vi "FromJSON.vi"(8 "error in (no error)":errorcluster, 10 "Request":string) -> (0 "error out":errorcluster, 3 "Request out":refnum<class "Request.lvclass">)   [LabVIEW 2015, in "Request.lvclass"]
uses:
  Request.lvclass
  JsonCluster.ctl
  Request.lvclass/Request.ctl
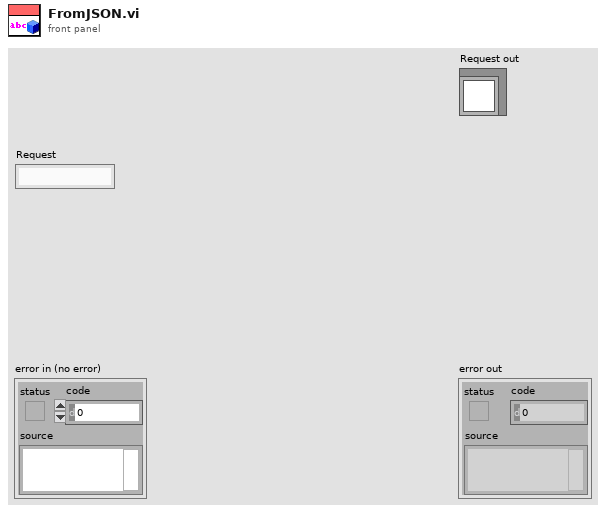
[diagram p1: front panel]
types:
  T1 = typedef "Request.lvclass/JsonCluster.ctl" = cluster{"RequestID":string, "PersonnelType":i32, "StartTime":string, "StartName":string, "AckTime":string, "AckName":string, "FulfilledTime":string, "FulfilledName":string, "Description":string, "RoomNumber":i32, "RequestType":i32, "Alarm":bool}
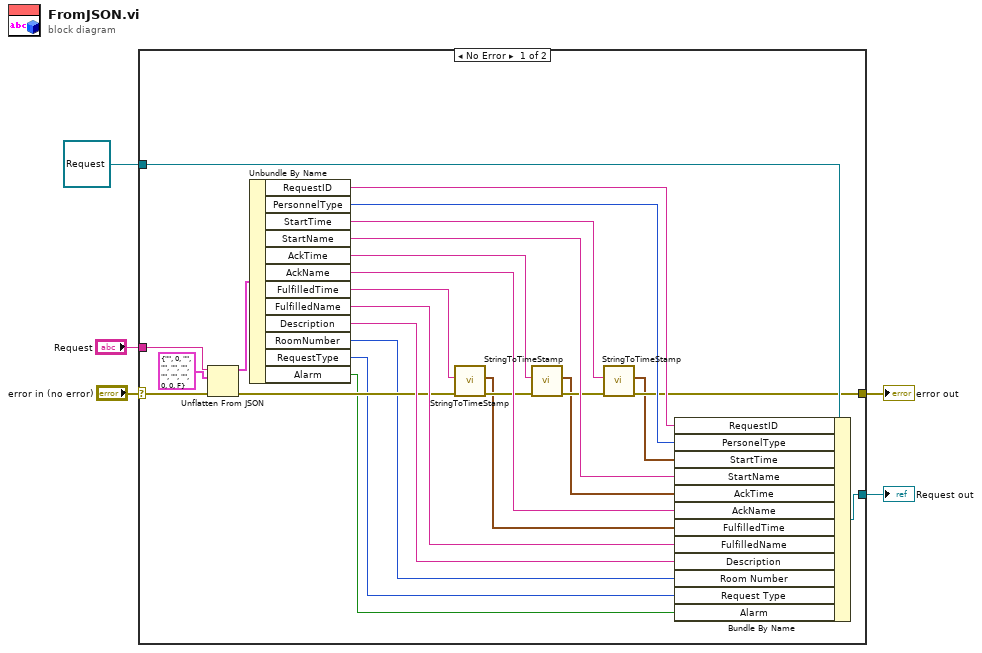
[diagram p0: block diagram]
diagram:
  n1 = case shown="No Error" "error in (no error)" {
    selector: "error in (no error)" -> [w16 w32]
    tunnel: [w17 w32] -> w4
    tunnel: [w29 w31] -> w2
    tunnel: refnum<class "Request.lvclass"> refnum ("Request in") -> [w30 w31]
    tunnel: "Request" -> [w28 _]
    frame No Error {
      n2 = Unflatten From JSON(JSON string=w28, type and defaults=T1 {"RequestID"="", "PersonnelType"=0, "StartTime"="", "StartName"="", "AckTime"="", "AckName"="", "FulfilledTime"="", "FulfilledName"="", "Description"="", "RoomNumber"=0, "RequestType"=0, "Alarm"=FALSE} ("RequestTable"), error in (no error)=w16) -> (value=w26:T1, error out=w15:errorcluster)  [unwired: 4 in]
      n3 = Unbundle By Name(w26) -> ("RequestID"=w25:string, "PersonnelType"=w20:i32, "StartTime"=w14:string, "StartName"=w21:string, "AckTime"=w12:string, "AckName"=w22:string, "FulfilledTime"=w10:string, "FulfilledName"=w23:string, "Description"=w24:string, "RoomNumber"=w8:i32, "RequestType"=w7:i32, "Alarm"=w6:bool)
      n4 = call "StringToTimeStamp.vi"("error in (no error)"=w15, "TimeStamp"=w10) -> ("error out"=w19:errorcluster, "Time Stamp"=w9:timestamp)  [unwired: 8 in]
      n5 = call "StringToTimeStamp.vi"("error in (no error)"=w19, "TimeStamp"=w12) -> ("error out"=w18:errorcluster, "Time Stamp"=w11:timestamp)  [unwired: 8 in]
      n6 = call "StringToTimeStamp.vi"("error in (no error)"=w18, "TimeStamp"=w14) -> ("error out"=w17:errorcluster, "Time Stamp"=w13:timestamp)  [unwired: 8 in]
      n7 = Bundle By Name(cluster=w30, "RequestID"=w25, "PersonelType"=w20, "StartTime"=w13, "StartName"=w21, "AckTime"=w11, "AckName"=w22, "FulfilledTime"=w9, "FulfilledName"=w23, "Description"=w24, "Room Number"=w8, "Request Type"=w7, "Alarm"=w6) -> (w29:refnum<class "Request.lvclass">)
    }
    frame Error {
    }
  }
  "error out" <- w4
  "Request out" <- w2
